vi "Byte stream to array - full frame.vi"(9 "Height":i32=2054, 10 "Width":i32=2456, 11 "u8Image":u8[](array[numeric])) -> (3 "Array":u16[][](array[numeric]))   [LabVIEW 2017]
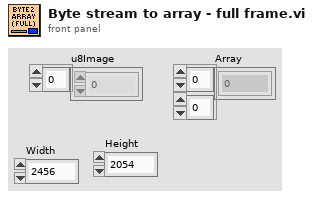
[diagram p1: front panel]
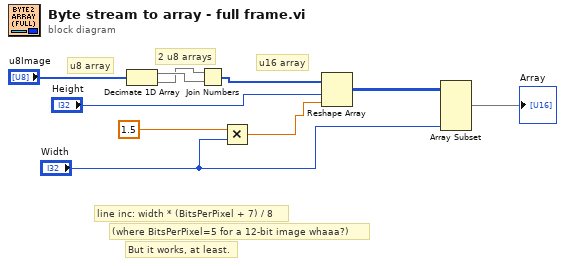
[diagram p0: block diagram]
diagram:
  # "But it works, at least."
  # "(where BitsPerPixel=5 for a 12-bit image whaaa?)"
  # "line inc: width * (BitsPerPixel + 7) / 8"
  # "u16 array"
  # "2 u8 arrays"
  # "u8 array"
  n1 = Decimate 1D Array("u8Image") -> (w8:u8[], w5:u8[])
  n2 = Join Numbers(hi=w5, lo=w8) -> ((hi.lo)=w9:u16[])
  n3 = Multiply(x=1.5, y="Width") -> (x*y=w3:dbl)
  n4 = Reshape Array(w9, "Height", w3) -> (w7:u16[][])
  n5 = Array Subset(array=w7, length (col)="Width") -> (→"Array":u16[][])  [unwired: 3 in]
